vi "HW_GEN - Write Module Channel Configurations.vi"(8 "error in":errorcluster caption="错误输入", 10 "ModCFG.CFG":T1[](array[typedef]), 11 "Path":path) -> (0 "error out":errorcluster caption="错误输出")   [LabVIEW 2016]
uses:
  Ctrls/HardWare _ Module Configuration.ctl
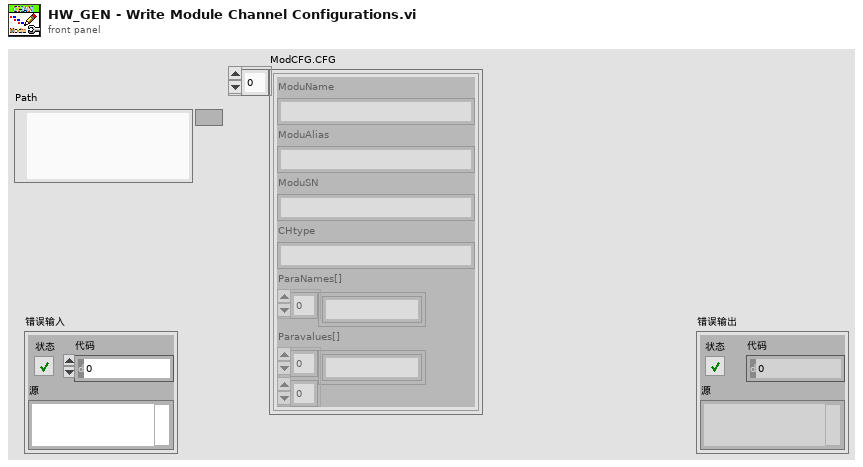
[diagram p1: front panel]
types:
  T1 = typedef "HardWare _ Module Configuration.ctl" = cluster{"ModuName":string, "ModuAlias":string, "ModuSN":string, "CHtype":string, "ParaNames[]":string[], "Paravalues[]":string[][]}
  T2 = enum16{"open", "replace", "create", "open or create", "replace or create", "replace or create with confirmation"}
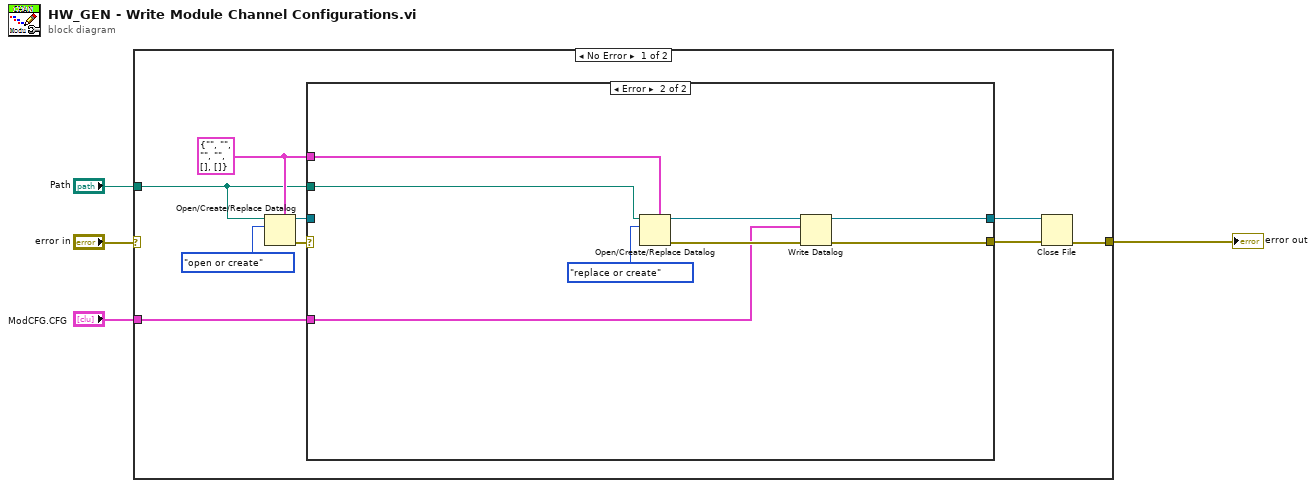
[diagram p0: block diagram]
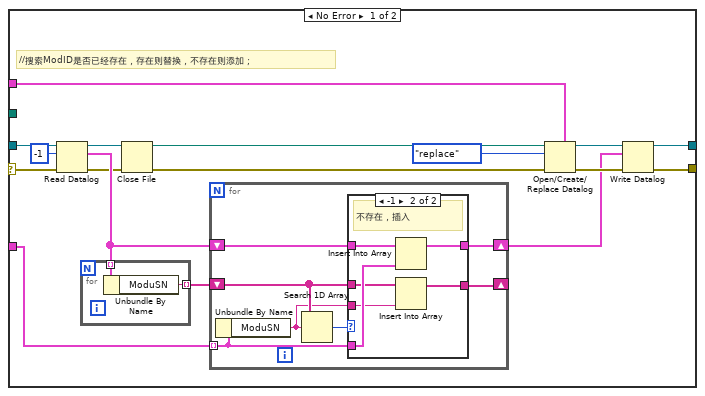
[diagram p2: hidden frame]
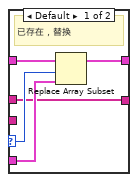
[diagram p3: hidden frame]
diagram:
  n1 = case shown="No Error" "error in" {
    selector: "error in" -> [_ w59]
    tunnel: [w5 w59] -> w1
    tunnel: "Path" -> [w8 _]
    tunnel: "ModCFG.CFG" -> [w13 _]
    frame No Error {
      w9 = T1 {"ModuName"="", "ModuAlias"="", "ModuSN"="", "CHtype"="", "ParaNames[]"=[], "Paravalues[]"=[]} ("ModuCfg")
      n2 = Open/Create/Replace Datalog(5:w9, 10:T2."open or create" ("操作(0:open)"), 11:w8) -> (0:w10:errorcluster, 3:w12:refnum<k1>)  [unwired: 3 in, 1 out]
      n3 = case shown="Error" w10 {
        selector: w10 -> [w25 _]
        tunnel: w13 -> [w27 w55]
        tunnel: [w20 w54] -> w6
        tunnel: w12 -> [w24 _]
        tunnel: w9 -> [w18 w53]
        tunnel: w8 -> [_ w52]
        tunnel: [w15 w51] -> w7
        frame No Error {
          # "//搜索ModID是否已经存在，存在则替换，不存在则添加；"
          n4 = Read Datalog(4:w25, 6:-1 ("总数(1)"), 7:w24) -> (0:w23:errorcluster, 2:w26:T1[], 3:w28:refnum<k1>)
          n5 = for {
            tunnel: w26 -> [w50] mode=indexing
            tunnel: [w49] -> w29 mode=indexing
            n6 = Unbundle By Name(w50) -> ("ModuSN"=w49:string)
          }
          n7 = Close File(refnum=w28, error in=w23) -> (path=w17:path, error out=w21:errorcluster)
          n8 = for {
            tunnel: w27 -> [w36] mode=indexing
            shift-right: [w34] -> w16
            shift-left: w26 -> [w35]
            shift-right: [w32] -> _
            shift-left: w29 -> [w33]
            n9 = Unbundle By Name(w36) -> ("ModuSN"=w31:string)
            n10 = Search 1D Array(1D array=w33, element=w31) -> (index of element=w37:i32)  [unwired: 1 in]
            n11 = case shown="-1" w37 {
              selector: w37 -> [w39 _]
              tunnel: w36 -> [w41 w47]
              tunnel: w35 -> [w42 w48]
              tunnel: [w40 w46] -> w34
              tunnel: w33 -> [w38 w45]
              tunnel: [w38 w44] -> w32
              tunnel: w31 -> [_ w43]
              frame Default {
                # "已存在，替换"
                n12 = Replace Array Subset(array=w42, new element=w41, index=w39) -> (w40:T1[])
              }
              frame -1 {
                # "不存在，插入"
                n13 = Insert Into Array(array=w48, new element=w47) -> (w46:T1[])  [unwired: 1 in]
                n14 = Insert Into Array(array=w45, new element=w43) -> (w44:string[])  [unwired: 1 in]
              }
            }
          }
          n15 = Open/Create/Replace Datalog(5:w18, 8:w21, 10:T2."replace" ("操作(0:open)"), 11:w17) -> (0:w22:errorcluster, 3:w19:refnum<k1>)  [unwired: 2 in, 1 out]
          n16 = Write Datalog(4:w22, 6:w16, 7:w19) -> (0:w20:errorcluster, 3:w15:refnum<k1>)
        }
        frame Error {
          n17 = Open/Create/Replace Datalog(5:w53, 10:T2."replace or create" ("操作(0:open)"), 11:w52) -> (0:w58:errorcluster, 3:w57:refnum<k1>)  [unwired: 3 in, 1 out]
          n18 = Write Datalog(4:w58, 6:w55, 7:w57) -> (0:w54:errorcluster, 3:w51:refnum<k1>)
        }
      }
      n19 = Close File(refnum=w7, error in=w6) -> (error out=w5:errorcluster)  [unwired: 1 out]
    }
    frame Error {
    }
  }
  "error out" <- w1
